vi "Get URI.vi"(11 "Unregister JSON in":refnum<class "Unregister JSON.lvclass">) -> (2 "URL":string, 3 "Unregister JSON out":refnum<class "Unregister JSON.lvclass">)   [LabVIEW 2020, in "wamplv.lvlib" / "Unregister JSON.lvclass"]
uses:
  Unregister JSON.lvclass
  Unregister JSON.lvclass/Unregister JSON.ctl
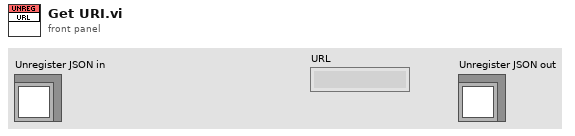
[diagram p1: front panel]
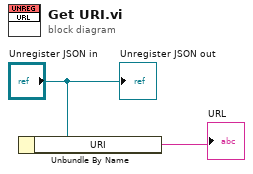
[diagram p0: block diagram]
diagram:
  n1 = Unbundle By Name("Unregister JSON in") -> ("URI"=→"URL":string)
  "Unregister JSON out" <- "Unregister JSON in"
